vi "BackOrderTraverse.vi"(6 "Stop Traverse":bool, 8 "error in":errorcluster caption="错误输入（无错误）", 9 "Data in":variant, 10 "vi reference":refnum<vi>, 11 "PanelLinkNode 输入":refnum<class "PanelLinkNode.lvclass"> caption="DNL_LabVIEW Object in") -> (0 "error out":errorcluster caption="错误输出", 1 "Data out":variant, 2 "vi reference out":refnum<vi>, 3 "PanelLinkNode 输出":refnum<class "PanelLinkNode.lvclass"> caption="DNL_LabVIEW Object out", 4 "Stop Traverse out":bool)   [LabVIEW 2016, in "PanelLinkNode.lvclass"]
uses:
  PanelLinkNode.lvclass
  PanelLinkNode.lvclass/PanelLinkNode.ctl
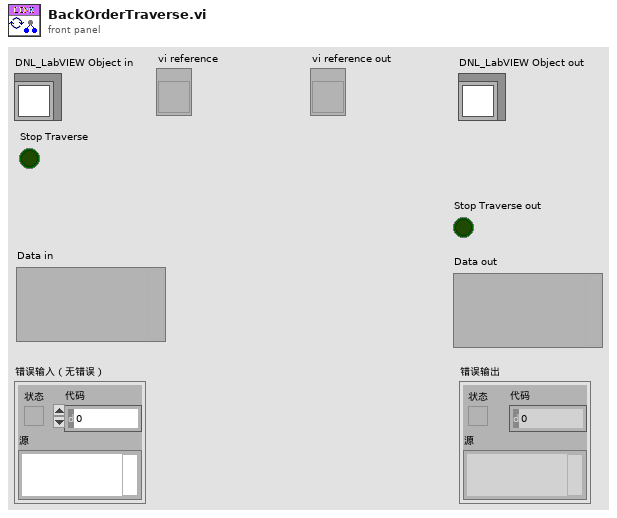
[diagram p1: front panel]
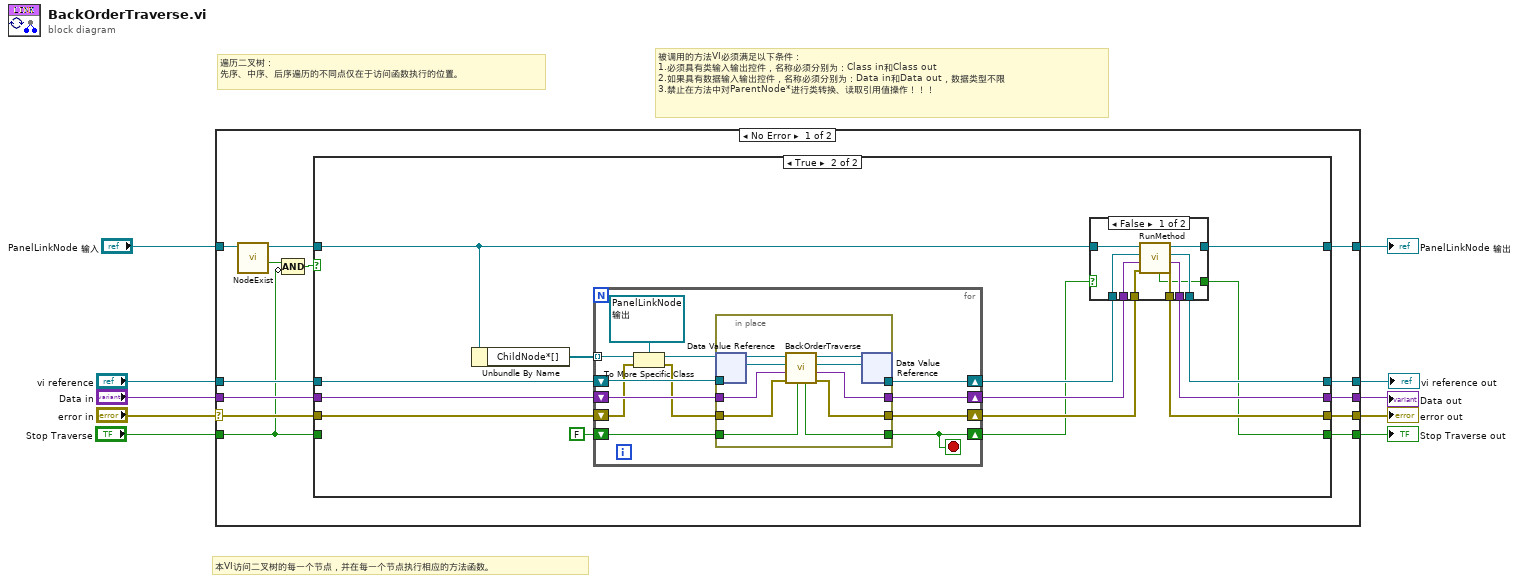
[diagram p0: block diagram]
diagram:
  # "遍历二叉树：\n先序、中序、后序遍历的不同点仅在于访问函数执行的位置。"
  # "本VI访问二叉树的每一个节点，并在每一个节点执行相应的方法函数。"
  # "被调用的方法VI必须满足以下条件：\n1.必须具有类输入输出控件，名称必须分别为：Class in和Class out\n2.如果具有数据输入输出控件，名称必须分别为：Data in和Data out，数据类型不限\n3.禁止在方法中对ParentNode*进行类转换、读取引用值操作！！！"
  n1 = case shown="No Error" "error in" {
    selector: "error in" -> [w13 w84]
    tunnel: [w17 w84] -> w9
    tunnel: [w23 w83] -> w7
    tunnel: "PanelLinkNode 输入" -> [w20 w83]
    tunnel: "Data in" -> [w21 w82]
    tunnel: "vi reference" -> [w22 w81]
    tunnel: [w18 w82] -> w5
    tunnel: [w16 w81] -> w1
    tunnel: "Stop Traverse" -> [w11 w80]
    tunnel: [w12 w80] -> w3
    frame No Error {
      n2 = call-dynamic "NodeExist.vi"("PanelLinkNode 输入"=w20) -> ("Node Exist?"=w15:bool, "PanelLinkNode 输出"=w19:refnum<class "PanelLinkNode.lvclass">)  [unwired: 8 in, 1 out]
      n3 = Compound Arithmetic op=AND(w15, invert w11) -> (w14:bool)
      n4 = case shown="True" w14 {
        tunnel: [w28 w40] -> w23
        tunnel: w22 -> [w26 w41]
        tunnel: w21 -> [w27 w43]
        tunnel: w19 -> [w28 w32]
        tunnel: [w27 w37] -> w18
        tunnel: [w25 w34] -> w17
        tunnel: [w26 w36] -> w16
        tunnel: w13 -> [w25 w42]
        tunnel: [w24 w30] -> w12
        tunnel: w11 -> [w24 _]
        frame False {
        }
        frame True {
          n5 = Unbundle By Name(w32) -> ("ChildNode*[]"=w33:refnum<data-value>[])
          n6 = for {
            tunnel: w33 -> [w68] mode=indexing
            shift-right: [w59] -> w35
            shift-left: w42 -> [w63]
            shift-right: [w60] -> w38
            shift-left: w43 -> [w65]
            shift-right: [w61] -> w39
            shift-left: w41 -> [w66]
            shift-right: [w58] -> w31
            shift-left: FALSE ("Stop Traverse out") -> [w62]
            stop <- w58 stop-if-true
            n7 = To More Specific Class(target class=refnum<data-value> refnum ("数据值引用"), reference=w68, error in=w63) -> (specific class reference=w67:refnum<data-value>, error out=w64:errorcluster)
            n8 = in-place {
              in-place-border: w66 -> [w77]
              in-place-border: w65 -> [w75]
              in-place-border: w64 -> [w73]
              in-place-border: w62 -> [w71]
              in-place-border: [w76] -> w61
              in-place-border: [w74] -> w60
              in-place-border: [w72] -> w59
              in-place-border: [w70] -> w58
              n9 = in-place-dvr #1(w67) -> (w79:refnum<class "PanelLinkNode.lvclass">)  [unwired: 1 out]
              n10 = call-dynamic "BackOrderTraverse.vi"("Stop Traverse"=w71, "error in"=w73, "Data in"=w75, "vi reference"=w77, "PanelLinkNode 输入"=w79) -> ("error out"=w72:errorcluster, "Data out"=w74:variant, "vi reference out"=w76:refnum<vi>, "PanelLinkNode 输出"=w78:refnum<class "PanelLinkNode.lvclass">, "Stop Traverse out"=w70:bool)  [unwired: 2 in]
              n11 = in-place-dvr #1(w78) -> ()  [unwired: 2 out]
            }
          }
          n12 = case shown="False" w31 {
            selector: w31 -> [_ w53]
            tunnel: [w52 w57] -> w40
            tunnel: w39 -> [w44 w55]
            tunnel: w38 -> [w51 w54]
            tunnel: [w50 w54] -> w37
            tunnel: [w49 w55] -> w36
            tunnel: w35 -> [w48 w56]
            tunnel: [w47 w56] -> w34
            tunnel: w32 -> [w46 w57]
            tunnel: [w45 w53] -> w30
            frame False {
              n13 = call-dynamic "RunMethod.vi"("error in (no error)"=w48, "Data in"=w51, "vi reference"=w44, "PanelLinkNode 输入"=w46) -> ("error out"=w47:errorcluster, "Data out"=w50:variant, "vi reference out"=w49:refnum<vi>, "PanelLinkNode 输出"=w52:refnum<class "PanelLinkNode.lvclass">, "Stop Traverse"=w45:bool)  [unwired: 3 in]
            }
            frame True {
            }
          }
        }
      }
    }
    frame Error {
    }
  }
  "error out" <- w9
  "PanelLinkNode 输出" <- w7
  "Data out" <- w5
  "Stop Traverse out" <- w3
  "vi reference out" <- w1
